vi "RT_mem_i40(SubVI).vi"(8 "Ini_val":dbl, 10 "start":bool, 11 "In":dbl format="%#_13g") -> (1 "output array":dbl[](array[numeric]))   [LabVIEW 2017]
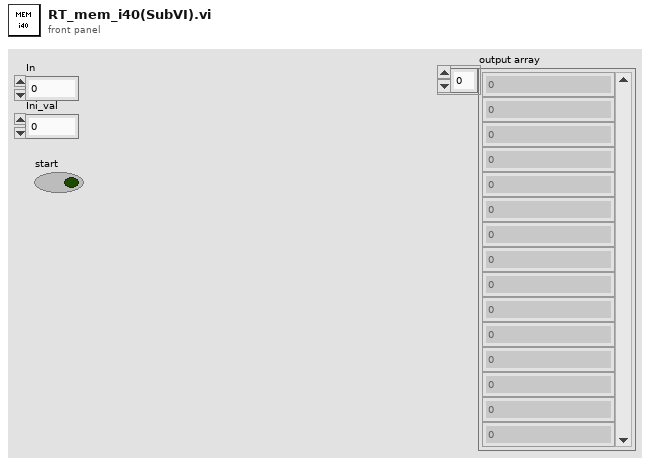
[diagram p1: front panel]
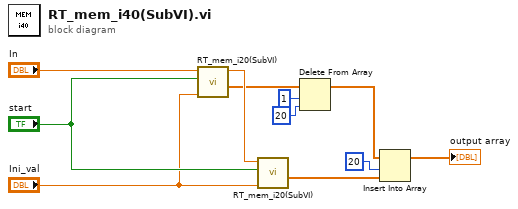
[diagram p0: block diagram]
diagram:
  n1 = call "RT_mem_i20(SubVI).vi"("Ini_val"="Ini_val", "start"="start", "In"="In") -> ("in_vec"=w4:dbl[], "in_i20"=w8:dbl)  [unwired: 7 in]
  n2 = call "RT_mem_i20(SubVI).vi"("Ini_val"="Ini_val", "start"="start", "In"=w8) -> ("in_vec"=w1:dbl[])  [unwired: 7 in, 1 out]
  n3 = Delete From Array(array=w4, length=1, index=20) -> (array with subset deleted=w3:dbl[])  [unwired: 1 out]
  n4 = Insert Into Array(array=w3, index=20, new element=w1) -> (→"output array":dbl[])
